vi "Untitled 3 (SubVI).vi"(9 "all rows":string[][](array[string]), 10 "Частота, Гц":dbl, 11 "XYGraph in":refnum<vi>) -> ()   [LabVIEW 2017]
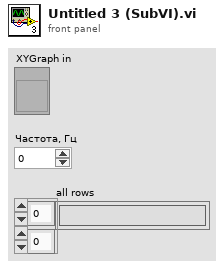
[diagram p1: front panel]
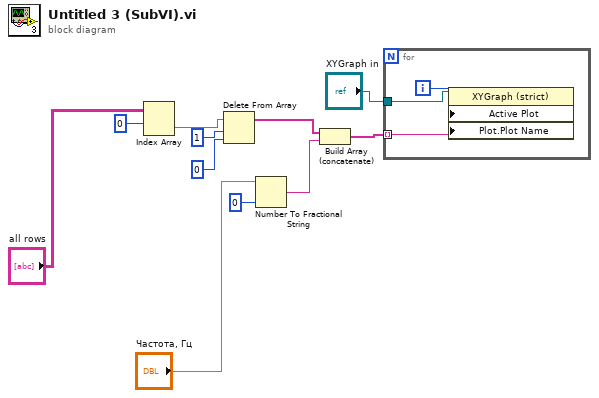
[diagram p0: block diagram]
diagram:
  n1 = Index Array(array="all rows", index (row)=0) -> (element=w4:string[])  [unwired: 1 in]
  n2 = Delete From Array(array=w4, length=1, index=0) -> (array with subset deleted=w7:string[])  [unwired: 1 out]
  n3 = Number To Fractional String(number="Частота, Гц", precision (6)=i16 0) -> (F-format string=w10:string)  [unwired: 2 in]
  n4 = Build Array (concatenate)(w7, w10) -> (w11:string[])
  n5 = for {
    tunnel: w11 -> [w13] mode=indexing
    tunnel: "XYGraph in" -> [w12]
    i -> [w14]
    n6 = property on="Property Node" class="XYGraph (strict)"(reference=w12, "Active Plot"=w14, "Plot.Plot Name"=w13) -> ()  [unwired: 1 in, 2 out]
  }
